vi "temporary.vi"() -> ()   [LabVIEW 2017]
uses:
  Error Handler/Controls/Error Data.ctl
  Error Handler/Controls/Error Level.ctl
  Configuration/Controls/Config Data Record.ctl
  Configuration/Controls/Config Command.ctl
  Controller/Controls/Elevator Location.ctl
panel:
  in  "Emergency":refnum<user-event>
  in  "Door Posit Change":refnum<user-event>
  in  "Direction Change":refnum<user-event>
  in  "Elapsed Time":refnum<data-value>
  in  "Location Change":refnum<user-event>
  in  "Location DVR":refnum<data-value>
  in  "Config CMD":refnum<user-event>
  in  "Data DVR":refnum<data-value>
  in  "Error":refnum<user-event>
  in  "Stop DVR":refnum<data-value>
  in  "Stop":refnum<user-event>
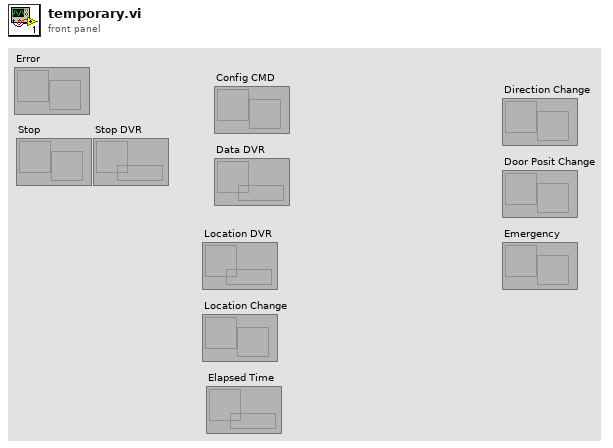
[diagram p1: front panel]
types:
  T1 = typedef "Elevator Location.ctl" = enum16{"1st Floor", "2nd Floor", "3rd Floor", "4th Floor"}
  T2 = typedef "Config Data Record.ctl" = cluster{"Door Open":dbl, "Door Close":dbl, "Travel Time":dbl, "Inactivity Time":dbl}
  T3 = typedef "Config Command.ctl" = enum16{"Read", "Update"}
  T4 = typedef "Error Data.ctl" = cluster{"Level":T5, "Source":enum16{"Display Console", "User Console"}, "Data":variant}
  T5 = typedef "Error Level.ctl" = enum16{"Console Error", "Sensor Interface IO Error", "Process Step Error"}
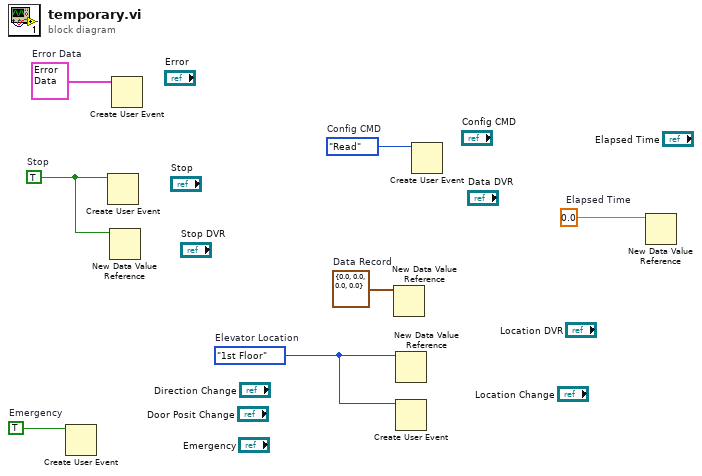
[diagram p0: block diagram]
diagram:
  w1 = TRUE  # Emergency
  w2 = 0.0  # Elapsed Time
  w3 = Elevator_Location."1st Floor"  # Elevator Location
  w4 = T2 {"Door Open"=0.0, "Door Close"=0.0, "Travel Time"=0.0, "Inactivity Time"=0.0}  # Data Record
  w5 = Config_Command."Read"  # Config CMD
  w6 = T4 {"Level"=enum."Console Error", "Source"=enum."Display Console", "Data"=variant}  # Error Data
  w7 = TRUE  # Stop
  n1 = Create User Event(user event datatype=w1) -> ()  [unwired: 1 in, 2 out]
  n2 = Create User Event(user event datatype=w7) -> ()  [unwired: 1 in, 2 out]
  n3 = New Data Value Reference(data value=w7) -> ()  [unwired: 1 in, 2 out]
  n4 = Create User Event(user event datatype=w6) -> ()  [unwired: 1 in, 2 out]
  n5 = New Data Value Reference(data value=w4) -> ()  [unwired: 1 in, 2 out]
  n6 = New Data Value Reference(data value=w3) -> ()  [unwired: 1 in, 2 out]
  n7 = Create User Event(user event datatype=w3) -> ()  [unwired: 1 in, 2 out]
  n8 = Create User Event(user event datatype=w5) -> ()  [unwired: 1 in, 2 out]
  n9 = New Data Value Reference(data value=w2) -> ()  [unwired: 1 in, 2 out]
